vi "Prepare Environment.vi"(8 "error in":errorcluster, 10 "Envrionment Options":T1, 11 "Paths":T2) -> (0 "error out":errorcluster, 3 "Environment out":refnum<k24>)   [LabVIEW 2024, in "WebView.lvclass"]
uses:
  WebView.lvclass
  <vilib>/sklein/WebView2/Libs/Microsoft.Web.WebView2.Core.dll
  Paths-cluster.ctl
  Core Envrionment Options--cluster.ctl
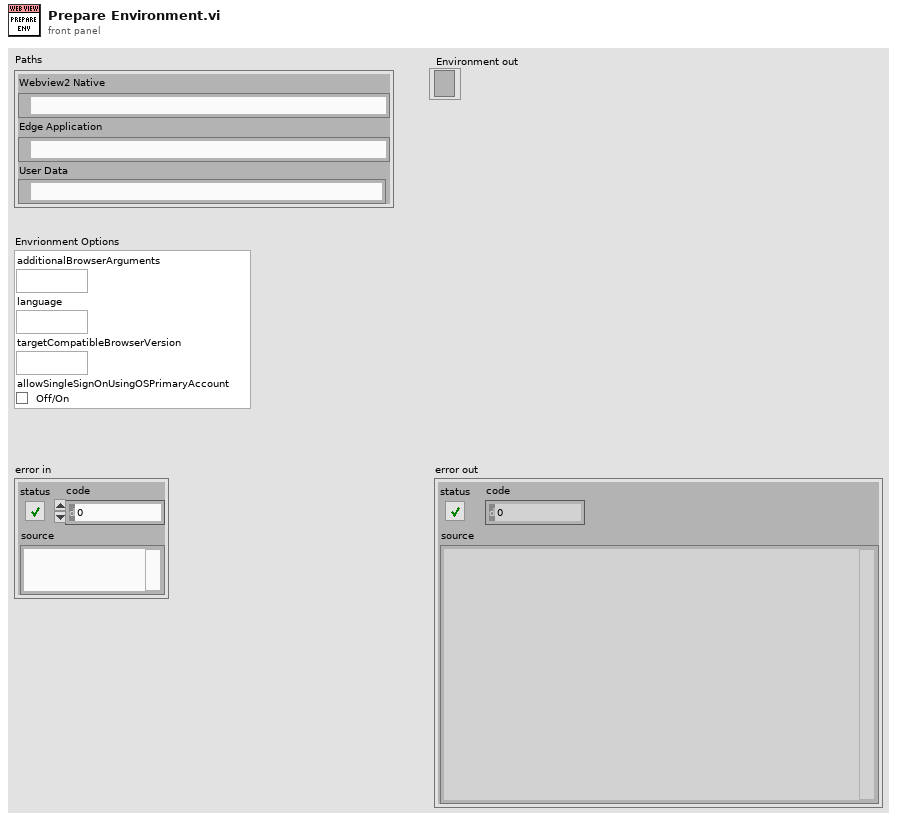
[diagram p1: front panel]
types:
  T1 = typedef "WebView.lvclass/Core Envrionment Options--cluster.ctl" = cluster{"additionalBrowserArguments":string, "language":string, "targetCompatibleBrowserVersion":string, "allowSingleSignOnUsingOSPrimaryAccount":bool}
  T2 = typedef "WebView.lvclass/Paths-cluster.ctl" = cluster{"Webview2 Native":path, "Edge Application":path, "User Data":path}
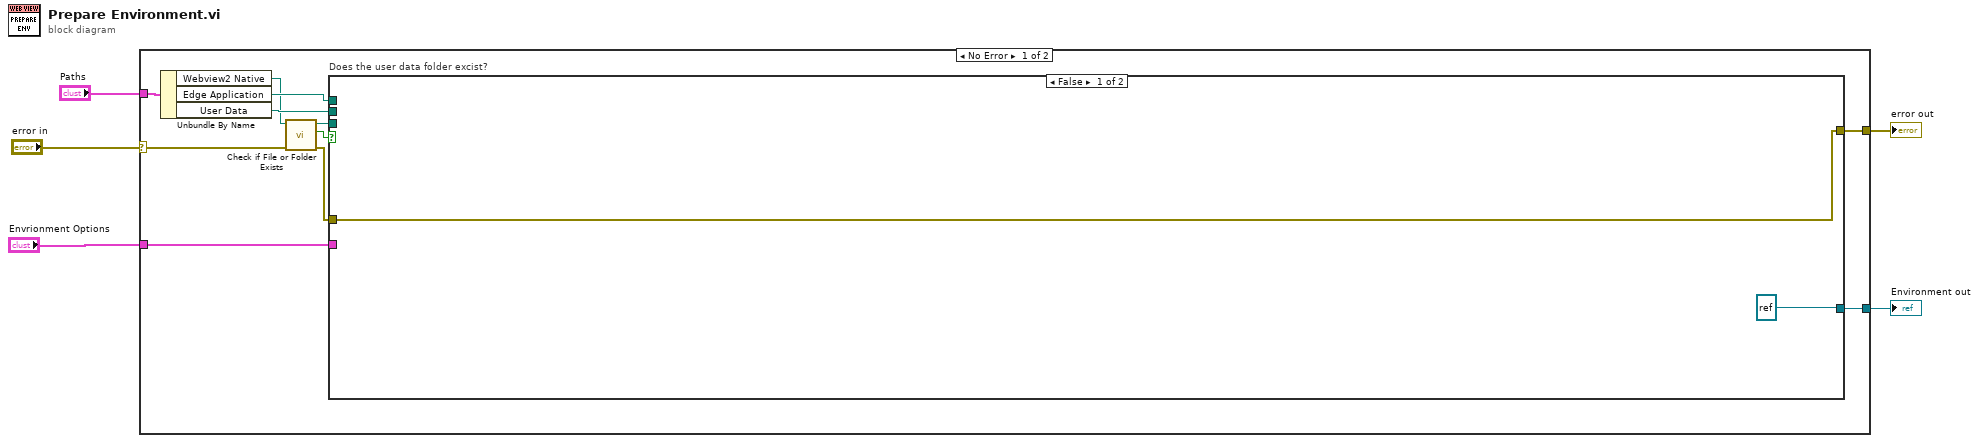
[diagram p0: block diagram]
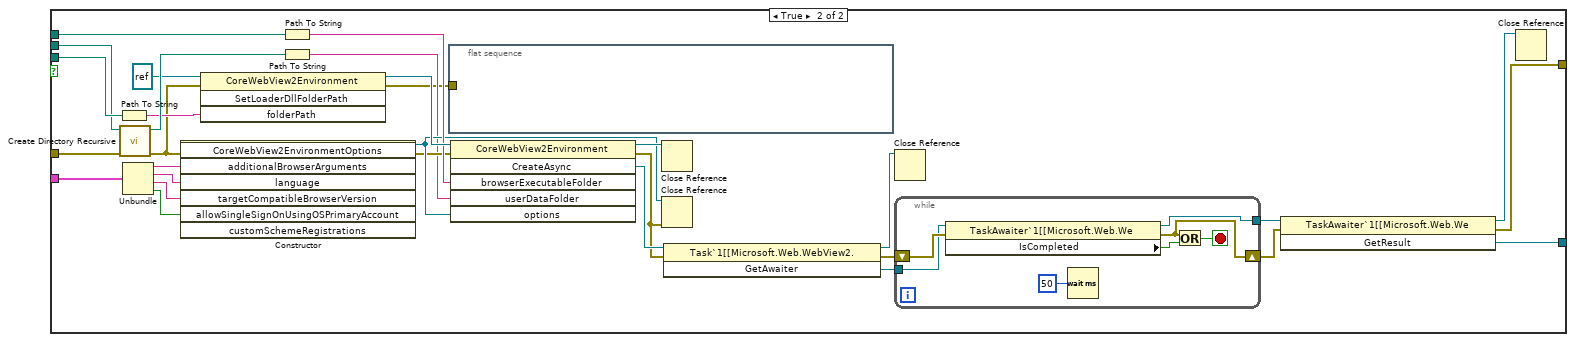
[diagram p2: hidden frame]
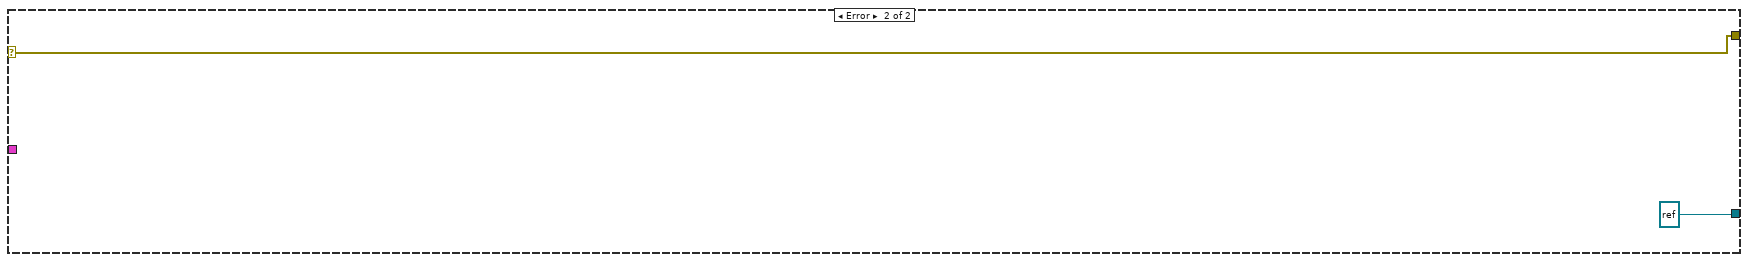
[diagram p3: hidden frame]
diagram:
  n1 = case shown="No Error" "error in" {
    selector: "error in" -> [w13 w57]
    tunnel: [w16 w57] -> w5
    tunnel: [w15 refnum<k24> refnum ("GetResult")] -> w4
    tunnel: "Paths" -> [w14 _]
    tunnel: "Envrionment Options" -> [w6 _]
    frame No Error {
      n2 = Unbundle By Name(w14) -> ("Webview2 Native"=w9:path, "Edge Application"=w12:path, "User Data"=w11:path)
      n3 = call <vilib>:"Check if File or Folder Exists.vi"("error in (no error)"=w13, "path"=w9) -> ("error out"=w10:errorcluster, "file or folder exists?"=w7:bool, "dup path"=w8:path)  [unwired: 7 in]
      n4 = case "Does the user data folder excist?" shown="False" w7 {
        tunnel: w12 -> [_ w45]
        tunnel: w11 -> [_ w39]
        tunnel: [refnum<k24> refnum ("GetResult") w20] -> w15
        tunnel: [w18 w35] -> w16
        tunnel: w10 -> [w18 w40]
        tunnel: w8 -> [_ w41]
        tunnel: w6 -> [_ w19]
        frame False {
        }
        frame True {
          n5 = Path To String(path=w41) -> (string=w25:string)
          n6 = call <vilib>:"Create Directory Recursive.vi"("error in (no error)"=w40, "directory"=w39) -> ("error out"=w23:errorcluster, "directory copy"=w28:path)  [unwired: 3 in, 1 out]
          n7 = Unbundle(w19) -> ("additionalBrowserArguments"=w34:string, "language"=w33:string, "targetCompatibleBrowserVersion"=w32:string, "allowSingleSignOnUsingOSPrimaryAccount"=w31:bool)
          n8 = constructor class="CoreWebView2EnvironmentOptions"(error in=w23, "additionalBrowserArguments"=w34, "language"=w33, "targetCompatibleBrowserVersion"=w32, "allowSingleSignOnUsingOSPrimaryAccount"=w31) -> (reference out=w30:refnum<k24>, error out=w29:errorcluster)  [unwired: 3 in, 6 out]
          n9 = invoke class="CoreWebView2Environment" method="SetLoaderDllFolderPath"(reference=refnum<k24> refnum ("environment"), error in=w23, "folderPath"=w25) -> (reference out=w48:refnum<k24>, error out=w24:errorcluster)  [unwired: 1 in, 2 out]
          n10 = Path To String(path=w45) -> (string=w47:string)
          n11 = Path To String(path=w28) -> (string=w27:string)
          n12 = flat-sequence {
            tunnel: w24 -> [_]
            frame #0 {
            }
          }
          n13 = invoke class="CoreWebView2Environment" method="CreateAsync"(reference=w48, error in=w29, "browserExecutableFolder"=w47, "userDataFolder"=w27, "options"=w30) -> (reference out=w37:refnum<k24>, error out=w21:errorcluster, "CreateAsync"=w46:refnum<k24>)  [unwired: 1 in, 3 out]
          n14 = Close Reference(reference=w37) -> ()  [unwired: 1 in, 1 out]
          n15 = Close Reference(reference=w30, error in (no error)=w21) -> ()  [unwired: 1 out]
          n16 = invoke class="Task`1[[Microsoft.Web.WebView2." method="GetAwaiter"(reference=w46, error in=w21) -> (reference out=w42:refnum<k24>, error out=w44:errorcluster, "GetAwaiter"=w22:refnum<k24>)  [unwired: 1 in]
          n17 = Close Reference(reference=w42) -> ()  [unwired: 1 in, 1 out]
          n18 = while {
            tunnel: w22 -> [w54]
            shift-right: [w49] -> w36
            shift-left: w44 -> [w55]
            tunnel: [w51] -> w43
            stop <- w50 stop-if-true
            n19 = property class="TaskAwaiter`1[[Microsoft.Web.We"(reference=w54, error in=w55) -> (reference out=w51:refnum<k24>, error out=w49:errorcluster, "IsCompleted"=w52:bool)
            n20 = Wait (ms)(milliseconds to wait=u32 50 ("millisecond multiple")) -> ()  [unwired: 1 out]
            n21 = Or(x=w49, y=w52) -> (x .or. y?=w50:bool)
          }
          n22 = invoke class="TaskAwaiter`1[[Microsoft.Web.We" method="GetResult"(reference=w43, error in=w36) -> (reference out=w38:refnum<k24>, error out=w35:errorcluster, "GetResult"=w20:refnum<k24>)  [unwired: 1 in]
          n23 = Close Reference(reference=w38) -> ()  [unwired: 1 in, 1 out]
        }
      }
    }
    frame Error {
    }
  }
  "error out" <- w5
  "Environment out" <- w4
